vi "test.vi"(9 "y":dbl[][](array[numeric]), 11 "Numeric":dbl) -> (0 "Numeric 2":dbl)   [LabVIEW 2013]
panel:
  out "String":string
  in  "Enum":enum16{"yes", "no"}(ring)
  out "replaced_string":string
  in  "save text?":bool
  out "dialogue indicator":dbl
  in  "dialogue?":bool
  out "2D":dbl[][](graph)
  out "1D":dbl[](graph)
  in  "Numeric 3":dbl
  out "Waveform Graph 2":dbl[](graph)
  out "Intensity Graph 2":dbl[][](graph)
  in  "Array 5":dbl[][](array[numeric])
  out "Cluster":cluster{"m disp":dbl, "n disp":dbl}
  in  "n":dbl
  in  "m":dbl
  in  "index":dbl
  out "result":dbl
  out "size":dbl
  out "Array 4":dbl[][](array[numeric])
  in  "Slide":dbl(slide) scale=0.0..100.0
  out "result":dbl
  in  "3":dbl
  in  "2":dbl
  in  "1":dbl
  out "Array 3":dbl[](array[numeric])
  in  "Array 2":dbl[][][](array[numeric])
  out "Array":dbl[](array[numeric])
  in  "delta_x":dbl
  in  "x0":dbl
  in  "stop":bool
  out "Waveform Graph":cluster{"x0":dbl, "delta_x":dbl, "y":dbl[][]}(graph)
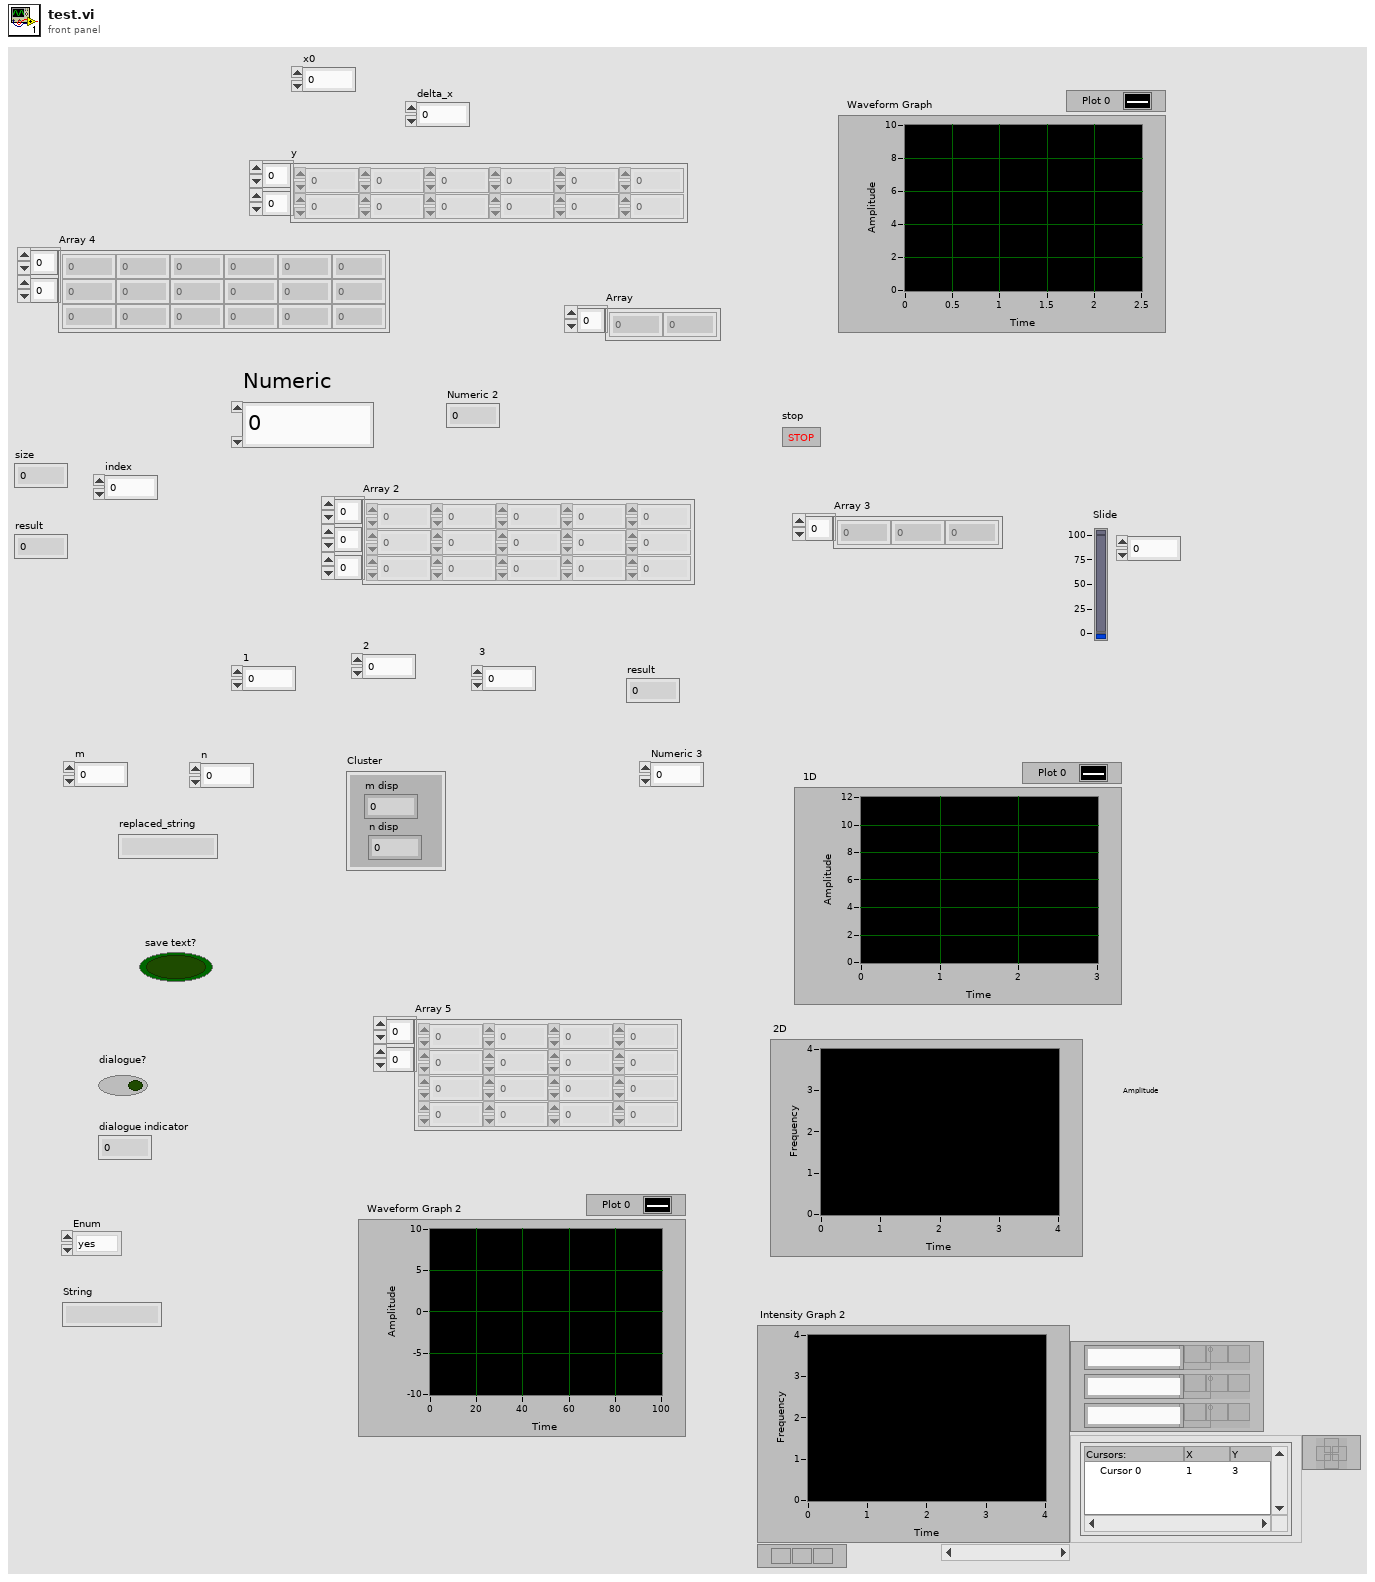
[diagram p1: front panel]
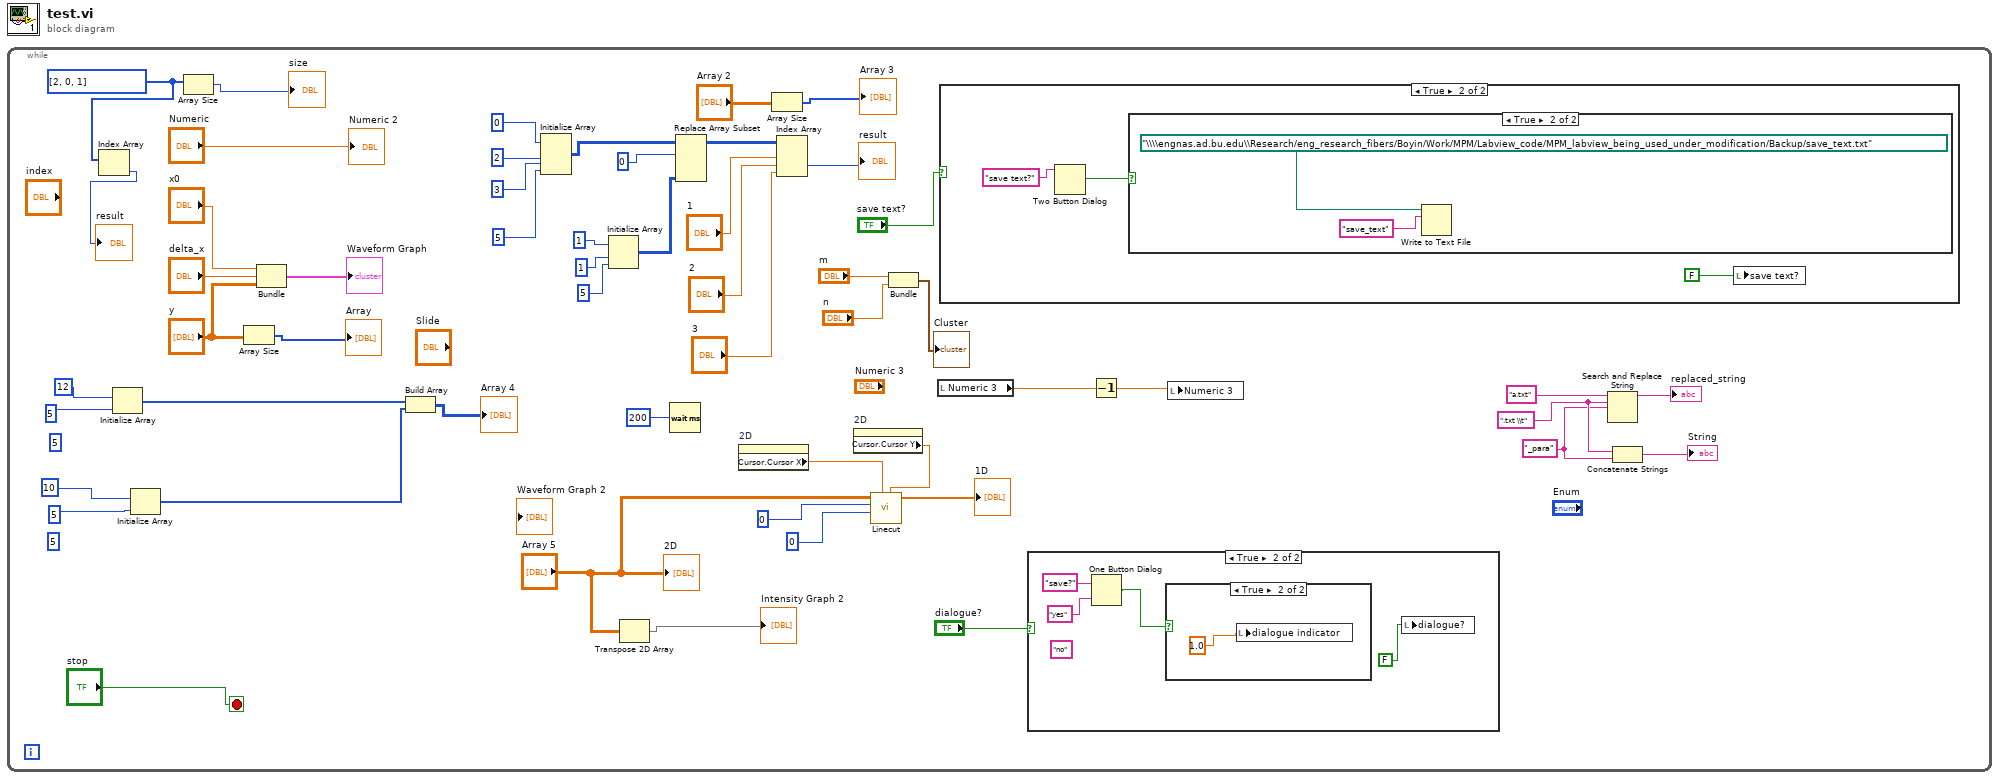
[diagram p0: block diagram]
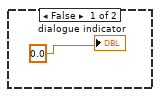
[diagram p5: hidden frame]
diagram:
  n1 = while {
    stop <- "stop" stop-if-true
    w2 = "_para"
    w3 = ".txt \\t"
    (unwired) 5
    (unwired) 5
    w28 = i32[] [2, 0, 1]
    n2 = Index Array(array=w28) -> (element=→"result":i32)  [unwired: 1 in]
    n3 = Initialize Array(12, 5) -> (w17:i32[])
    n4 = Initialize Array(10, 5) -> (w16:i32[])
    n5 = Array Size(array=w28) -> (size(s)=→"size":i32)
    n6 = Array Size(array="y") -> (size(s)=→"Array":i32[])
    n7 = Bundle("x0"="x0", "delta_x"="delta_x", "y"="y") -> (→"Waveform Graph":cluster{"x0":dbl, "delta_x":dbl, "y":dbl[][]})  [unwired: 1 in]
    n8 = Build Array(w17, w16) -> (→"Array 4":i32[][])
    n9 = Initialize Array(0, 2, 3, 5) -> (w39:i32[][][])
    n10 = Initialize Array(1, 1, 5) -> (w37:i32[][])
    n11 = Transpose 2D Array(2D array="Array 5") -> (transposed array=→"Intensity Graph 2":dbl[][])
    n12 = Wait (ms)(milliseconds to wait=200) -> ()  [unwired: 1 out]
    n13 = Replace Array Subset(array=w39, new element=w37, index (dim 0)=0) -> (w36:i32[][][])  [unwired: 2 in]
    n14 = property on="2D" class="IntGraph (strict)"() -> ("Cursor.Cursor X"=w10:dbl)  [unwired: 2 in, 2 out]
    n15 = Array Size(array="Array 2") -> (size(s)=→"Array 3":i32[])
    n16 = Index Array(array=w36, index (dim 0)="1", index (dim 1)="2", index (dim 2)="3") -> (element=→"result":i32)
    n17 = property on="2D" class="IntGraph (strict)"() -> ("Cursor.Cursor Y"=w9:dbl)  [unwired: 2 in, 2 out]
    n18 = call "Linecut.vi"("linecut y position"=w9, "linecut x position"=w10, "Linear/Log"=0, "Linecut direction (fast/slow)"=0, "Input image"="Array 5") -> ("Linecut profile"=→"1D":dbl[])  [unwired: 5 in, 1 out]
    n19 = Bundle("m"="m", "n"="n") -> (→"Cluster":cluster{"m":dbl, "n":dbl})  [unwired: 1 in]
    n20 = local read "Numeric 3"() -> (w22:dbl)
    n21 = case shown="True" "save text?" {
      frame False {
      }
      frame True {
        n22 = Two Button Dialog(message="save text?") -> (T button?=w57:bool)  [unwired: 2 in]
        n23 = case shown="True" w57 {
          frame False {
          }
          frame True {
            n24 = Write to Text File(file (use dialog)=path "\\\\engnas.ad.bu.edu\\Research/eng_research_fibers/Boyin/Work/MPM/Labview_code/MPM_labview_being_used_under_modification/Backup/save_text.txt", text="save_text") -> ()  [unwired: 2 in, 3 out]
          }
        }
        n25 = local write "save text?"(FALSE) -> ()
      }
    }
    n26 = case shown="True" "dialogue?" {
      frame False {
      }
      frame True {
        (unwired) "no"
        n27 = One Button Dialog(message="save?", button name ("OK")="yes") -> (true=w61:bool)
        n28 = case shown="True" w61 {
          frame False {
            "dialogue indicator" <- 0.0
          }
          frame True {
            n29 = local write "dialogue indicator"(1.0) -> ()
          }
        }
        n30 = local write "dialogue?"(FALSE) -> ()
      }
    }
    n31 = Decrement(x=w22) -> (x-1=w23:dbl)
    n32 = local write "Numeric 3"(w23) -> ()
    n33 = Search and Replace String(input string="a.txt", search string=w3, replace string=w2) -> (result string=→"replaced_string":string)  [unwired: 5 in, 3 out]
    n34 = Concatenate Strings(w3, w2) -> (→"String":string)
    "Numeric 2" <- "Numeric"
    "2D" <- "Array 5"
  }
